vi "RGB2gray.vi"(11 "引用句柄输入":T1) -> (3 "引用句柄输出":T1)   [LabVIEW 2013]
doc: "本VI用于将RGB图像信号转化为灰度图像信号，操作上直接输入RGB信号引用即可输出grayscale图像引用。"
uses:
  <vilib>/vision/Image Controls.llb/IMAQ Image.ctl
  <vilib>/vision/NI_Vision_Development_Module.lvlib
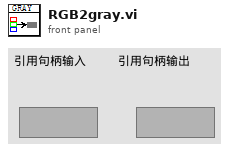
[diagram p1: front panel]
types:
  T1 = typedef "IMAQ Image.ctl" = refnum<image>
  T2 = typedef "Image Type" = u32
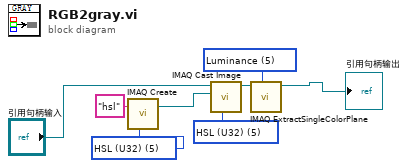
[diagram p0: block diagram]
diagram:
  w5 = 5 items=["Red", "Green", "Blue", "Hue", "Saturation", "Luminance", "Value", "Intensity"] ("Color Plane")
  w3 = T2 5 items=["Grayscale (U8)", "Grayscale (I16)", "Grayscale (SGL)", "Complex (CSG)", "RGB (U32)", "HSL (U32)", "RGB (U64)"] ("Image Type")
  w7 = T2 5 items=["Grayscale (U8)", "Grayscale (I16)", "Grayscale (SGL)", "Complex (CSG)", "RGB (U32)", "HSL (U32)", "RGB (U64)"] ("Image Type")
  n1 = call "IMAQ Create"("Image Name"="hsl", "Image Type"=w7) -> ("New Image"=w1:T1)  [unwired: 3 in, 1 out]
  n2 = call "IMAQ Cast Image"("Image Type"=w3, "Image Dst"=w1, "Image Src"="引用句柄输入") -> ("Image Dst Out"=w4:T1)  [unwired: 7 in, 1 out]
  n3 = call "IMAQ ExtractSingleColorPlane"("Color Plane"=w5, "Image Src"=w4) -> ("Image Dst Out"=→"引用句柄输出":T1)  [unwired: 8 in, 1 out]
